vi "winkelabhängige_linie_zeichnen.vi"(6 "Linienlänge":sgl, 9 "Angle":sgl, 10 "x":sgl, 11 "y":sgl) -> ()   [LabVIEW 2014]
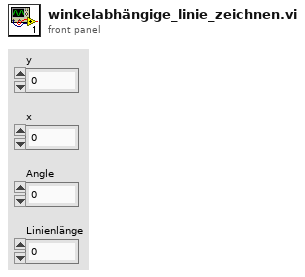
[diagram p1: front panel]
types:
  T1 = cluster{"[0]":cluster{"x":sgl, "y":sgl}, "[1]":cluster{"x":sgl, "y":sgl}, "[2]":cluster{"x":sgl, "y":sgl}, "[3]":cluster{"x":sgl, "y":sgl}, "[4]":cluster{"x":sgl, "y":sgl}, "[5]":cluster{"x":sgl, "y":sgl}, "[6]":cluster{"x":sgl, "y":sgl}, "[7]":cluster{"x":sgl, "y":sgl}, "[8]":cluster{"x":sgl, "y":sgl}}
  T2 = typedef "IMAQ Image.ctl" = refnum<image>
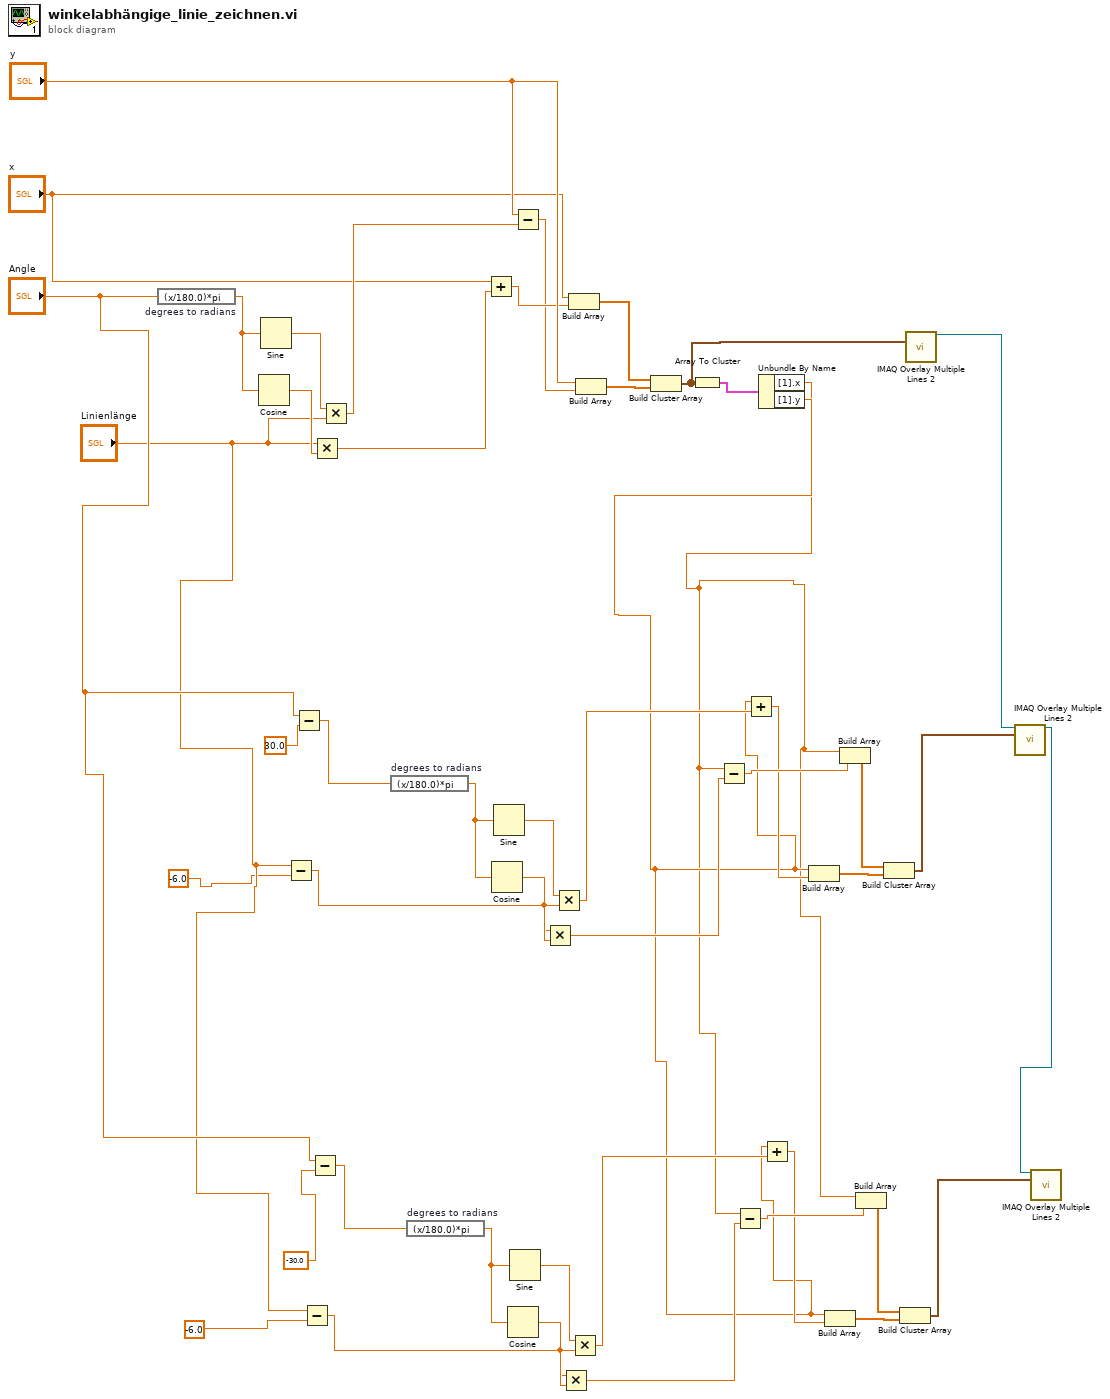
[diagram p0: block diagram]
diagram:
  n1 = expression code="(x/180.0)*pi" "degrees to radians"("Angle") -> (w40:sgl)
  n2 = Cosine(x=w40) -> (cos(x)=w39:sgl)
  n3 = Sine(x=w40) -> (sin(x)=w38:sgl)
  n4 = Subtract(x="Linienlänge", y=sgl -6.0) -> (x-y=w27:sgl)
  n5 = Subtract(x="Angle", y=sgl 30.0) -> (x-y=w28:sgl)
  n6 = Subtract(x="Linienlänge", y=sgl -6.0) -> (x-y=w12:sgl)
  n7 = Subtract(x="Angle", y=sgl -30.0) -> (x-y=w13:sgl)
  n8 = Multiply(x="Linienlänge", y=w39) -> (x*y=w47:sgl)
  n9 = Multiply(x=w38, y="Linienlänge") -> (x*y=w48:sgl)
  n10 = expression code="(x/180.0)*pi" "degrees to radians"(w28) -> (w31:sgl)
  n11 = expression code="(x/180.0)*pi" "degrees to radians"(w13) -> (w16:sgl)
  n12 = Add(x="x", y=w47) -> (x+y=w44:sgl)
  n13 = Cosine(x=w31) -> (cos(x)=w30:sgl)
  n14 = Sine(x=w31) -> (sin(x)=w29:sgl)
  n15 = Cosine(x=w16) -> (cos(x)=w15:sgl)
  n16 = Sine(x=w16) -> (sin(x)=w14:sgl)
  n17 = Subtract(x="y", y=w48) -> (x-y=w43:sgl)
  n18 = Multiply(x=w27, y=w30) -> (x*y=w36:sgl)
  n19 = Multiply(x=w29, y=w27) -> (x*y=w37:sgl)
  n20 = Multiply(x=w12, y=w15) -> (x*y=w21:sgl)
  n21 = Build Array("x", w44) -> (w41:sgl[])
  n22 = Multiply(x=w14, y=w12) -> (x*y=w22:sgl)
  n23 = Build Array("y", w43) -> (w42:sgl[])
  n24 = Build Cluster Array(w41, w42) -> (w23:cluster{"x":sgl, "y":sgl}[])
  n25 = Array To Cluster(array=w23) -> (cluster=w25:T1)
  n26 = Unbundle By Name(w25) -> ("[1].x"=w7:sgl, "[1].y"=w8:sgl)
  n27 = Subtract(x=w7, y=w36) -> (x-y=w35:sgl)
  n28 = Subtract(x=w7, y=w21) -> (x-y=w20:sgl)
  n29 = Add(x=w8, y=w37) -> (x+y=w34:sgl)
  n30 = Add(x=w8, y=w22) -> (x+y=w19:sgl)
  n31 = Build Array(w8, w34) -> (w33:sgl[])
  n32 = Build Array(w8, w19) -> (w18:sgl[])
  n33 = Build Array(w7, w35) -> (w32:sgl[])
  n34 = Build Array(w7, w20) -> (w17:sgl[])
  n35 = Build Cluster Array(w32, w33) -> (w26:cluster{"x":sgl, "y":sgl}[])
  n36 = Build Cluster Array(w17, w18) -> (w11:cluster{"x":sgl, "y":sgl}[])
  n37 = call "IMAQ Overlay Multiple Lines 2"("Line End Points"=w23) -> ("Image"=w1:T2, "Image Out"=w24:T2)  [unwired: 12 in, 1 out]
  n38 = call "IMAQ Overlay Multiple Lines 2"("Image"=w24, "Line End Points"=w26) -> ("Image Out"=w6:T2)  [unwired: 12 in, 1 out]
  n39 = call "IMAQ Overlay Multiple Lines 2"("Image"=w6, "Line End Points"=w11) -> ()  [unwired: 12 in, 2 out]
